vi "Device Not Found Error.vi"(8 "error in":errorcluster, 11 "Config in":refnum<class "Config.lvclass">) -> (0 "error out":errorcluster, 3 "Config out":refnum<class "Config.lvclass">)   [LabVIEW 2023, in "Config.lvlib" / "Config.lvclass"]
uses:
  Config.lvclass
  Config.lvclass/Config.ctl
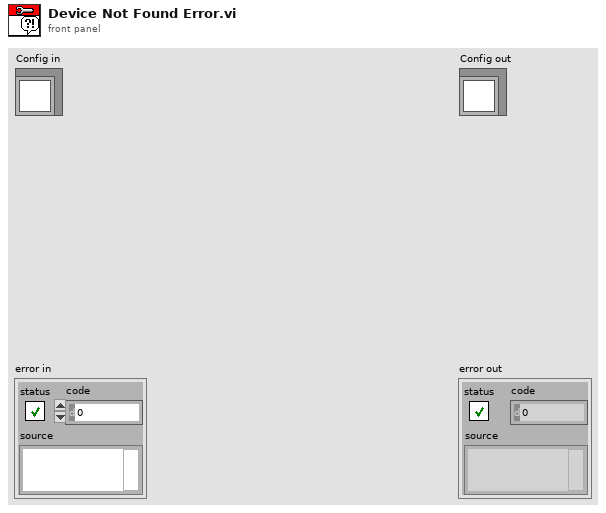
[diagram p1: front panel]
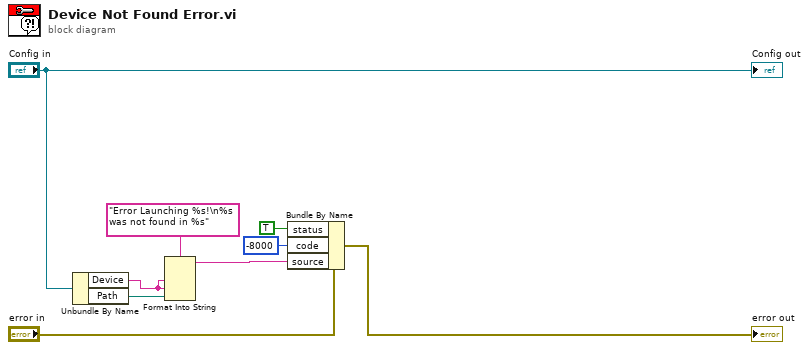
[diagram p0: block diagram]
diagram:
  n1 = Unbundle By Name("Config in") -> ("Device"=w1:string, "Path"=w2:path)
  n2 = Format Into String(format string="Error Launching %s!\n%s was not found in %s", w1, w1, w2) -> (resulting string=w4:string)  [unwired: 2 in, 1 out]
  n3 = Bundle By Name(cluster="error in", "status"=TRUE, "code"=-8000, "source"=w4) -> (→"error out":errorcluster)
  "Config out" <- "Config in"
